vi "Handle Last Ack Core.vi"(4 "error in (no error)":errorcluster, 6 "Last Ack":refnum<class "Last Ack.lvclass">, 7 "CS++RTMainActor in":refnum<class "CS++RTMainActor.lvclass">) -> (0 "error out":errorcluster, 3 "CS++RTMainActor out":refnum<class "CS++RTMainActor.lvclass">)   [LabVIEW 2014, in "CS++RTMain.lvlib" / "CS++RTMainActor.lvclass"]
doc: "(<B>Filename</B>: Actor Framework.lvlib:Actor.lvclass:Handle Last Ack Core.vi)\n\nDefines how the caller actor responds to the Last Ack message from a nested actor. The Last Ack message is the final message a nested actor sends to its caller before it shuts down. The message contains information about the final state of the nested actor.\n\nBy default, this method does nothing except return any error the nested actor sent. A descendant class may override this method to define behavior."
uses:
  CS++RTMainActor.lvclass
  <vilib>/ActorFramework/LastAck/Last Ack.lvclass
  <vilib>/ActorFramework/LastAck/Last Ack.lvclass/Last Ack.ctl
  CS++RTClasses/CS++RTMessageLogger/CS++RTMessageLogger.lvclass
  <vilib>/ActorFramework/Actor/Actor.lvclass
  CSPP_Core/Classes/CS++BaseClasses/MessageLogger/CS++MessageLogger.lvclass
  CSPP_Core/Libraries/Utilities/CS++Utilities.lvlib
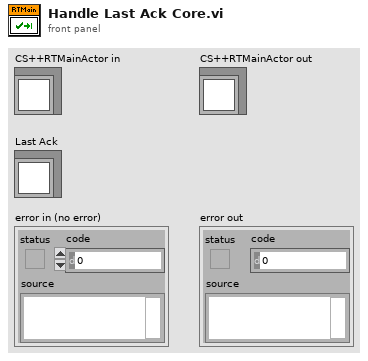
[diagram p1: front panel]
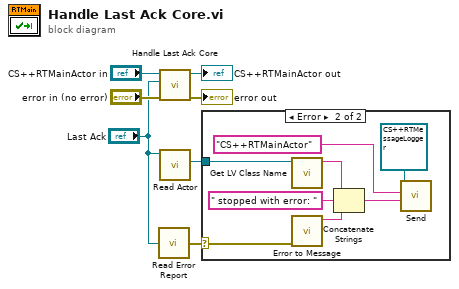
[diagram p0: block diagram]
diagram:
  n1 = call <vilib>:"Read Error Report.vi"("Last Ack"="Last Ack") -> ("error report"=w1:errorcluster)
  n2 = call-parent "Handle Last Ack Core.vi"("error in (no error)"="error in (no error)", "Last Ack"="Last Ack", "Actor in"="CS++RTMainActor in") -> ("error out"=→"error out":errorcluster, "Actor out"=→"CS++RTMainActor out":refnum<class "CS++RTMainActor.lvclass">)  [unwired: 3 in]
  n3 = call <vilib>:"Read Actor.vi"("Last Ack"="Last Ack") -> ("Actor"=w2:refnum<class "Actor.lvclass">)  [unwired: 10 in]
  n4 = case shown="Error" w1 {
    selector: w1 -> [_ w12]
    tunnel: w2 -> [_ w15]
    frame No Error {
    }
    frame Error {
      n5 = call <vilib>:"Get LV Class Name.vi"("object"=w15) -> ("class name"=w14:string)  [unwired: 9 in, 1 out]
      n6 = call "Error to Message.vi"("Error In"=w12) -> ("Error Message"=w11:string)  [unwired: 9 in, 1 out]
      n7 = Concatenate Strings(w14, " stopped with error: " ("string"), w11) -> (w10:string)
      n8 = call "Send.vi"("Message Content"=w10, "Message Tag"="CS++RTMainActor" ("String to write"), "CS++MessageLogger in"=refnum<class "CS++RTMessageLogger.lvclass"> refnum ("CS++RTClasses.lvlib:CS++RTMessageLogger.lvclass")) -> ()  [unwired: 7 in, 2 out]
    }
  }
